vi "FGV.vi"(8 "error in":errorcluster, 10 "name":string, 11 "Action":enum16{"Create", "Get", "Destroy"}(ring)=enum."Destroy") -> (0 "error out":errorcluster, 3 "Queue out":refnum<queue>)   [LabVIEW 2018]
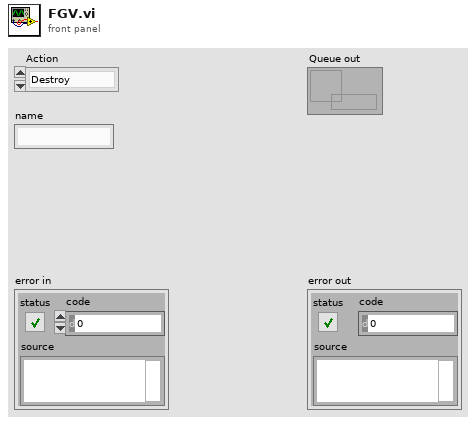
[diagram p1: front panel]
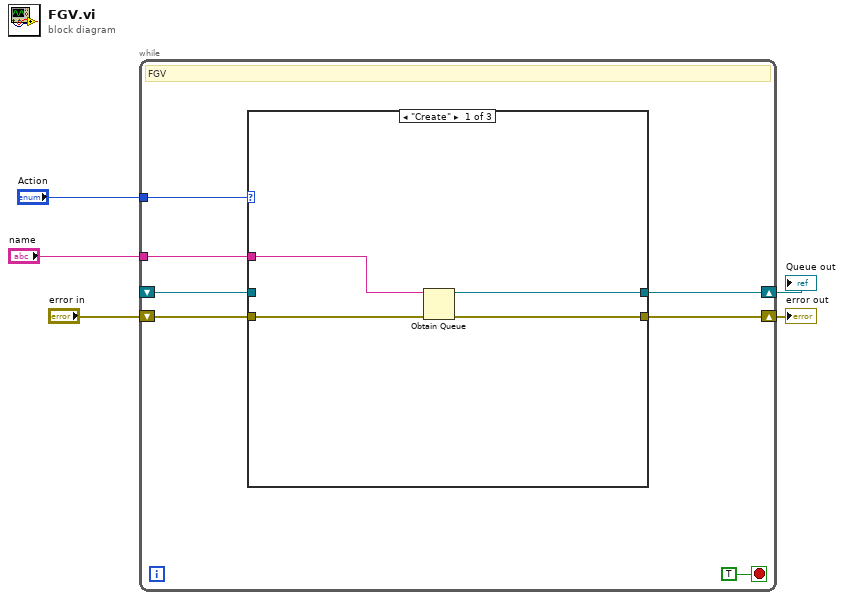
[diagram p0: block diagram]
diagram:
  n1 = while {
    tunnel: "Action" -> [w12]
    shift-right: [w9] -> w3
    shift-left: "error in" -> [w8]
    shift-right: [w10] -> w5
    shift-left: _ -> [w7]
    tunnel: "name" -> [w6]
    stop <- TRUE stop-if-true
    # "FGV"
    n2 = case shown="\"Create\"" w12 {
      tunnel: [w16 w18 _] -> w10
      tunnel: [w15 w17 _] -> w9
      tunnel: w8 -> [w14 w17 _]
      tunnel: w7 -> [_ w18 _]
      tunnel: w6 -> [w13 _ _]
      frame "Create" {
        n3 = Obtain Queue(name (unnamed)=w13, error in (no error)=w14) -> (queue out=w16:refnum<queue>, error out=w15:errorcluster)  [unwired: 3 in, 1 out]
      }
      frame "Get", Default {
      }
      frame "Destroy" {
      }
    }
  }
  "error out" <- w3
  "Queue out" <- w5
